vi "Execute.vi"(8 "error in (no error)":errorcluster, 10 "command":string, 11 "PQ Connection in":refnum<class "PQ Connection.lvclass">) -> (0 "error out":errorcluster, 1 "PQ Result  out":refnum<class "PQ Result.lvclass">, 3 "PQ Connection out":refnum<class "PQ Connection.lvclass">, 4 "PGresult":T1)   [LabVIEW 2015, in "PQ Connection.lvclass"]
uses:
  PQ Connection.lvclass
  Result/PQ Result.lvclass
  <vilib>/LAVA/libpq/Types/PGresult.ctl
  PQ Connection.lvclass/PQ Connection.ctl
  Result/PQ Result.lvclass/PQ Result.ctl
  <vilib>/LAVA/_libpq_internal_deps/libpq.dll
  <vilib>/LAVA/libpq/__lava_libpq.lvlib
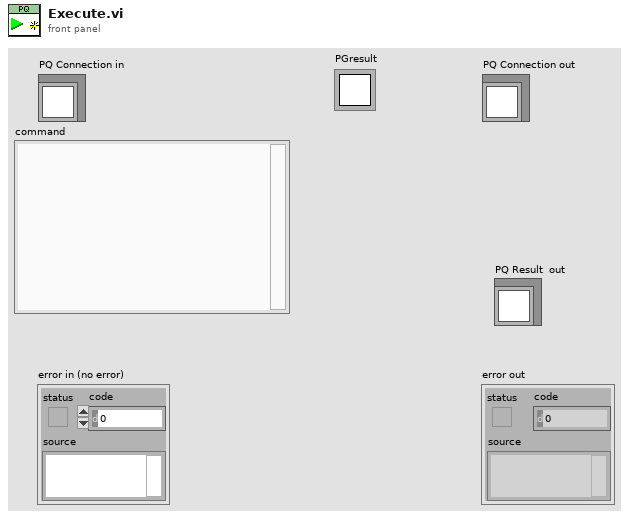
[diagram p1: front panel]
types:
  T1 = typedef "__lava_libpq.lvlib/PGresult.ctl" = refnum<k1>
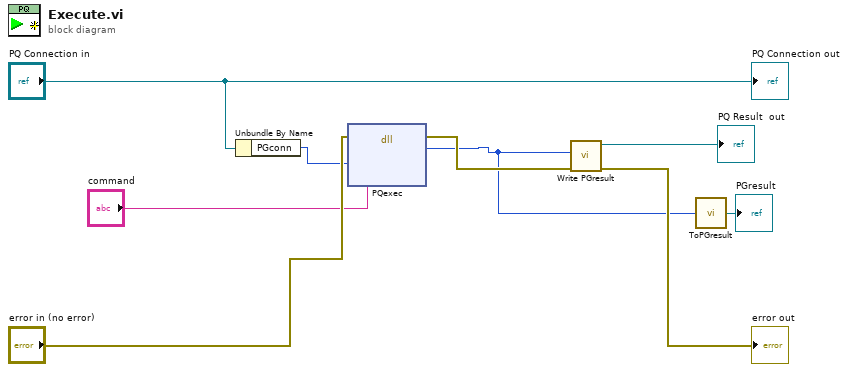
[diagram p0: block diagram]
diagram:
  n1 = Unbundle By Name("PQ Connection in") -> ("PGconn"=w7:u32)
  n2 = dll-call lib="C:/Program Files (x86)/National Instruments/LabVIEW 2015/vi.lib/LAVA/_libpq_internal_deps/libpq.dll" fn="PQexec"(error in="error in (no error)", "PGconn"=w7, "command"="command") -> (error out=w6:errorcluster, "PQresult"=w2:u32)  [unwired: 4 in, 1 out]
  n3 = call "Write PGresult.vi"("error in (no error)"=w6, "PGresult"=w2) -> ("error out"=→"error out":errorcluster, "PQ Result  out"=→"PQ Result  out":refnum<class "PQ Result.lvclass">)  [unwired: 8 in]
  n4 = call <vilib>:"ToPGresult.vi"("PGconn_ptr"=w2) -> ("PGresult"=→"PGresult":T1)
  "PQ Connection out" <- "PQ Connection in"
